vi "ex4 another.vi"() -> ()   [LabVIEW 2019]
panel:
  out "Boolean":bool
  in  "bp1":bool
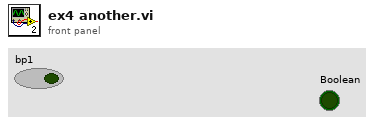
[diagram p1: front panel]
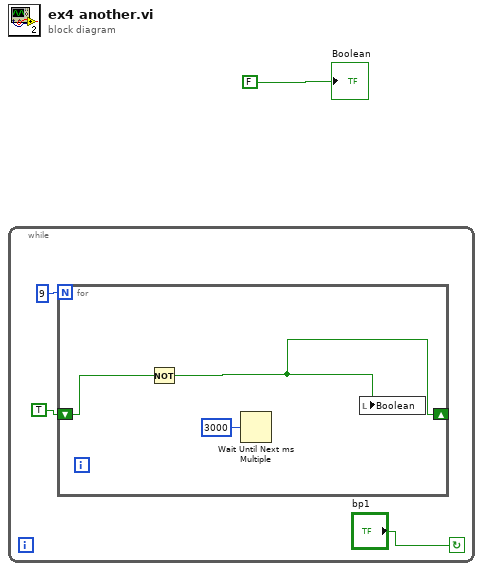
[diagram p0: block diagram]
diagram:
  n1 = while {
    stop <- "bp1" continue-if-true
    n2 = for {
      N: 9 -> [_]
      shift-right: [w6] -> _
      shift-left: TRUE -> [w7]
      n3 = Not(x=w7) -> (.not. x?=w6:bool)
      n4 = Wait Until Next ms Multiple(millisecond multiple=u32 3000) -> ()  [unwired: 1 out]
      n5 = local write "Boolean"(w6) -> ()
    }
  }
  "Boolean" <- FALSE
